vi "Do 8-Contact Sample Hall Calculations.vi"(8 "error in (no error)":errorcluster) -> (0 "error out":errorcluster)   [LabVIEW 2016, in "Hall Effect Library.lvlib"]
uses:
  Hall Effect Library.lvlib
  Global Variables/Hall Effect Data.vi
  Global Variables/Test Settings.vi
panel:
  out "uH":dbl
  out "Rh":dbl
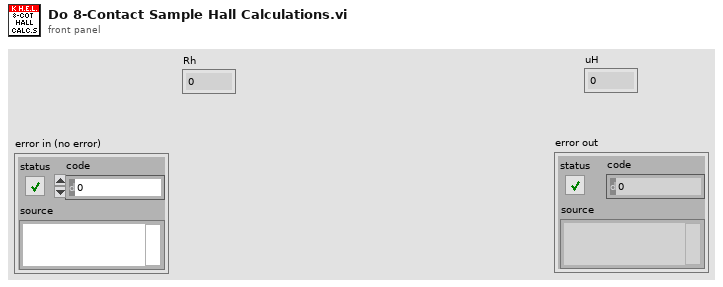
[diagram p1: front panel]
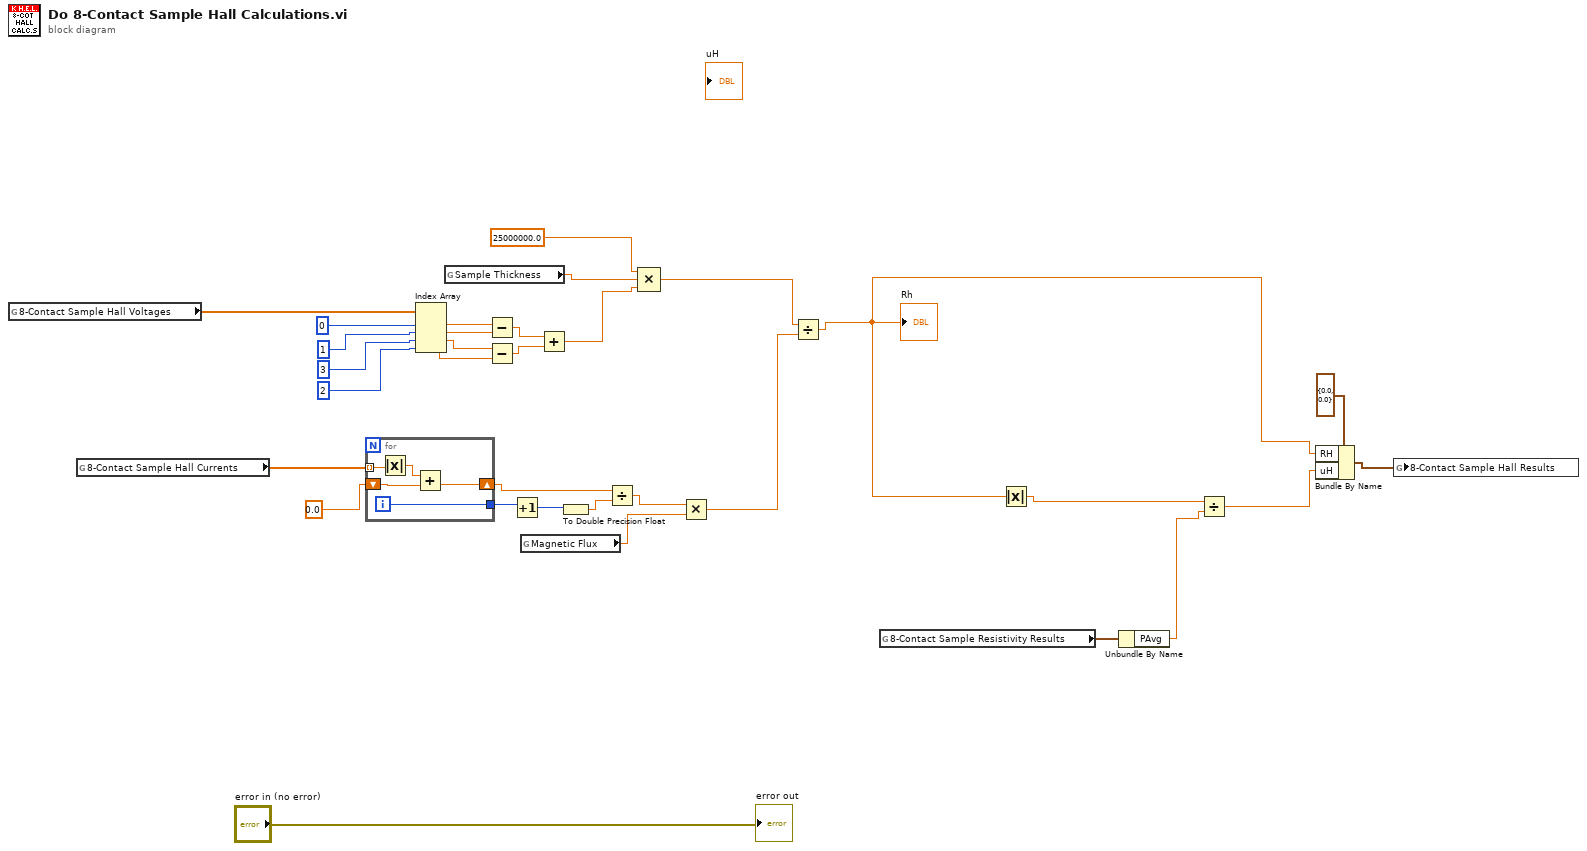
[diagram p0: block diagram]
diagram:
  n1 = global read "Hall Effect Data.vi" "8-Contact Sample Hall Voltages"() -> (w14:dbl[])
  n2 = global read "Hall Effect Data.vi" "8-Contact Sample Hall Currents"() -> (w30:dbl[])
  n3 = for {
    shift-right: [w36] -> w26
    shift-left: 0.0 -> [w37]
    tunnel: w30 -> [w34] mode=indexing
    tunnel: [w35] -> w29
    i -> [w35]
    n4 = Absolute Value(x=w34) -> (abs(x)=w33:dbl)
    n5 = Add(x=w33, y=w37) -> (x+y=w36:dbl)
  }
  n6 = Index Array(array=w14, index #1=0, index #2=1, index #3=3, index #4=2) -> (element #1=w21:dbl, element #2=w20:dbl, element #3=w19:dbl, element #4=w18:dbl)
  n7 = global read "Test Settings.vi" "Sample Thickness"() -> (w13:dbl)
  n8 = Subtract(x=w21, y=w20) -> (x-y=w17:dbl)
  n9 = Subtract(x=w19, y=w18) -> (x-y=w16:dbl)
  n10 = Increment(x=w29) -> (x+1=w28:i32)
  n11 = global read "Test Settings.vi" "Magnetic Flux"() -> (w10:dbl)
  n12 = Add(x=w17, y=w16) -> (x+y=w15:dbl)
  n13 = To Double Precision Float(number=w28) -> (double precision float=w27:dbl)
  n14 = Divide(x=w26, y=w27) -> (x/y=w11:dbl)
  n15 = Compound Arithmetic op=MULTIPLY(25000000.0, w13, w15) -> (w9:dbl)
  n16 = Multiply(x=w11, y=w10) -> (x*y=w8:dbl)
  n17 = Divide(x=w9, y=w8) -> (x/y=w2:dbl)
  "Rh" <- w2
  n18 = global read "Hall Effect Data.vi" "8-Contact Sample Resistivity Results"() -> (w7:cluster{"PAvg":dbl, "PA":dbl, "PB":dbl})
  n19 = Absolute Value(x=w2) -> (abs(x)=w1:dbl)
  n20 = Unbundle By Name(w7) -> ("PAvg"=w6:dbl)
  n21 = Divide(x=w1, y=w6) -> (x/y=w4:dbl)
  n22 = Bundle By Name(cluster=cluster{"RH":dbl, "uH":dbl} {"RH"=0.0, "uH"=0.0} ("8-Contact Sample Hall Results"), "RH"=w2, "uH"=w4) -> (w3:cluster{"RH":dbl, "uH":dbl})
  n23 = global write "Hall Effect Data.vi" "8-Contact Sample Hall Results"(w3) -> ()
  "error out" <- "error in (no error)"
